vi "Insight_Select_Upgrade.vi"(8 "error in (no error)":errorcluster, 10 "IP address":string, 11 "telnet connection":T1) -> (0 "error out":errorcluster, 3 "telnet  connection out":T1)   [LabVIEW 2015]
uses:
  Telnet Session.ctl
panel:
  out "disconnect error":errorcluster
  out "status":bool
  in  "Laser Search":enum32{"Available Upgrades", "Upgrading"}(tab)
  in  "select":bool
  in  "Available Upgrades":i32(listbox)
  in  "cancel":bool
  out "Upgrade Indicator":cluster{u8, u8}(slide)={0, 49} caption="Search Indicator" scale=0.0..100.0
  # "Upgrading laser..."
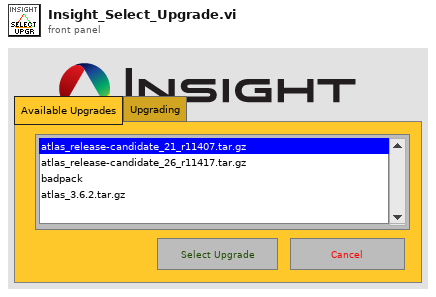
[diagram p1: front panel]
types:
  T1 = typedef "Telnet Session.ctl" = refnum<k1>
  T2 = enum32{"Invalid", "Default", "Floating", "Floating/Auto-Hide", "Modal"}
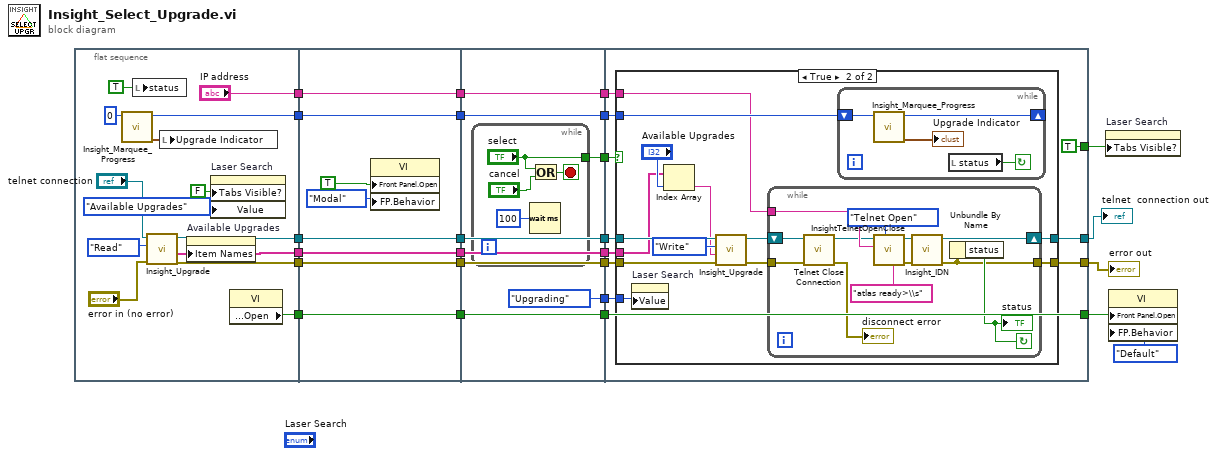
[diagram p0: block diagram]
diagram:
  n1 = flat-sequence {
    tunnel: [w31] -> w22
    tunnel: [w34] -> w17
    tunnel: [w33] -> w14
    tunnel: [w29] -> w11
    tunnel: ["IP address"] -> w6
    tunnel: [w26] -> w2
    tunnel: w22 -> [w45]
    tunnel: [w45] -> w23
    tunnel: [w44] -> w18
    tunnel: w17 -> [w44]
    tunnel: [w43] -> w15
    tunnel: w14 -> [w43]
    tunnel: [w42] -> w12
    tunnel: w11 -> [w42]
    tunnel: [w41] -> w7
    tunnel: w6 -> [w41]
    tunnel: [w40] -> w3
    tunnel: w2 -> [w40]
    tunnel: w23 -> [w55]
    tunnel: [w55] -> w21
    tunnel: [w54] -> w20
    tunnel: [w53] -> w19
    tunnel: w18 -> [w53]
    tunnel: [w52] -> w16
    tunnel: w15 -> [w52]
    tunnel: [w51] -> w13
    tunnel: w12 -> [w51]
    tunnel: [w50] -> w8
    tunnel: w7 -> [w50]
    tunnel: [w49] -> w4
    tunnel: w3 -> [w49]
    tunnel: [enum32{"Available Upgrades", "Upgrading"}."Upgrading" ("Laser Search")] -> w1
    tunnel: [w70] -> w24
    tunnel: w21 -> [w70]
    tunnel: w20 -> [w69]
    tunnel: w19 -> [w68]
    tunnel: w16 -> [w67]
    tunnel: w13 -> [w66]
    tunnel: [w65] -> w10
    tunnel: [w64] -> w9
    tunnel: w8 -> [w63]
    tunnel: [TRUE ("Tabs Visible?")] -> w5
    tunnel: w4 -> [w61]
    tunnel: w1 -> [w60]
    frame #0 {
      n2 = call "Insight_Marquee_Progress.vi"("x"=u8 0) -> ("Progress Indicator"=w38:cluster{u8, u8}, "x (out)"=w29:u8)  [unwired: 9 in]
      n3 = local write "status"(TRUE ("status")) -> ()
      n4 = call "Insight_Upgrade.vi"("error in (no error)"="error in (no error)", "Mode (Read / Write)"=enum8{"Write", "Read"}."Read", "telnet connection"="telnet connection") -> ("error out"=w33:errorcluster, "upgrade files"=w26:string[], "telnet  connection out"=w34:T1)  [unwired: 5 in, 1 out]
      n5 = local write "Upgrade Indicator"(w38) -> ()
      n6 = property on="Available Upgrades" class="LstBox (strict)"("Item Names"=w26) -> ()  [unwired: 2 in, 2 out]
      n7 = property on="Laser Search" class="TabCtl (strict)"("Tabs Visible?"=FALSE, "Value"=enum32{"Available Upgrades", "Upgrading"}."Available Upgrades" ("Laser Search")) -> ()  [unwired: 2 in, 2 out]
      n8 = property class="VI"() -> ("Front Panel.Open"=w31:bool)  [unwired: 2 in, 2 out]
    }
    frame #1 {
      n9 = property class="VI"("Front Panel.Open"=TRUE ("Front Panel Window:Open"), "FP.Behavior"=T2."Modal" ("Front Panel Window:Behavior")) -> ()  [unwired: 2 in, 2 out]
    }
    frame #2 {
      n10 = while {
        tunnel: ["select"] -> w54
        stop <- w57 stop-if-true
        n11 = Wait (ms)(milliseconds to wait=u32 100) -> ()  [unwired: 1 out]
        n12 = Or(x="select", y="cancel") -> (x .or. y?=w57:bool)
      }
    }
    frame #3 {
      n13 = case shown="True" w69 {
        tunnel: w68 -> [w71 w85]
        tunnel: w67 -> [w72 w84]
        tunnel: w66 -> [_ w80]
        tunnel: [w72 w76] -> w65
        tunnel: [w71 w77] -> w64
        tunnel: w63 -> [_ w75]
        tunnel: w61 -> [_ w74]
        tunnel: w60 -> [_ w73]
        frame False {
        }
        frame True {
          n14 = property on="Laser Search" class="TabCtl (strict)"("Value"=w73) -> ()  [unwired: 2 in, 2 out]
          n15 = Index Array(array=w74, index="Available Upgrades") -> (element=w81:string)
          n16 = call "Insight_Upgrade.vi"("error in (no error)"=w84, "filename"=w81, "Mode (Read / Write)"=enum8{"Write", "Read"}."Write", "telnet connection"=w85) -> ("error out"=w78:errorcluster, "telnet  connection out"=w79:T1)  [unwired: 4 in, 2 out]
          n17 = while {
            shift-right: [w90] -> w77
            shift-left: w79 -> [w89]
            tunnel: w75 -> [w96]
            tunnel: w78 -> [w88]
            tunnel: [w91] -> w76
            stop <- w92 continue-if-true
            n18 = call "Telnet Close Connection.vi"("error in (no error)"=w88, "telnet connection"=w89) -> ("error out"=→"disconnect error":errorcluster, "telnet connection out"=w87:T1)  [unwired: 8 in]
            n19 = call "InsightTelnetOpenClose.vi"("telnet connection"=w87, "IP Address"=w96, "Method"=enum16{"Telnet Open", "Telnet Close"}."Telnet Open", "line separator"="atlas ready>\\s") -> ("telnet connection"=w94:T1, "error out"=w93:errorcluster)  [unwired: 5 in]
            n20 = call "Insight_IDN.vi"("error in (no error)"=w93, "telnet connection"=w94) -> ("error out"=w91:errorcluster, "telnet  connection out"=w90:T1)  [unwired: 7 in, 1 out]
            n21 = Unbundle By Name(w91) -> ("status"=w92:bool)
            "status" <- w92
          }
          n22 = while {
            shift-right: [w100] -> _
            shift-left: w80 -> [w101]
            stop <- w98 continue-if-true
            n23 = call "Insight_Marquee_Progress.vi"("x"=w101) -> ("Progress Indicator"=→"Upgrade Indicator":cluster{u8, u8}, "x (out)"=w100:u8)  [unwired: 9 in]
            n24 = local read "status"() -> (w98:bool)
          }
        }
      }
    }
  }
  n25 = property on="Laser Search" class="TabCtl (strict)"("Tabs Visible?"=w5) -> ()  [unwired: 2 in, 2 out]
  n26 = property class="VI"("Front Panel.Open"=w24, "FP.Behavior"=T2."Default" ("Front Panel Window:Behavior")) -> ()  [unwired: 2 in, 2 out]
  "telnet  connection out" <- w9
  "error out" <- w10
